vi "from string.vi"(8 "error in":errorcluster, 9 "data":string, 10 "version":string, 11 "user tag bus module configuration In":refnum<class "user tag bus module configuration.lvclass">) -> (0 "error out":errorcluster, 3 "user tag bus module configuration Out":refnum<class "user tag bus module configuration.lvclass">)   [LabVIEW 2013, in "user tag bus module configuration.lvclass"]
doc: "Provides an interface for loading a module configuration from a file or other serialized data source. It is recommended that all children of this class store data in two sets--data required for its own initialization, and any data required for parent initialization--and that each implementation uses the <b>Call Parent Method</b> primitive to de-serialize parent information. As a result, it is expected that every module configuration class calls <b>component configuration.lvclass:From String.vi</b>."
uses:
  user tag bus module configuration.lvclass
  state module configuration.ctl
  <vilib>/NI/Tag Bus Module Framework/channel/TBM channel.lvclass
  control module configuration.ctl
  gains.ctl
  <vilib>/NI/Tag Bus Module Framework/module configuration/TBM module configuration.lvclass
  user tag bus module configuration.lvclass/user tag bus module configuration.ctl
  <vilib>/NI/Tag Bus Module Framework/root configuration/wrap data.vi
  <vilib>/NI/Tag Bus Module Framework/root configuration/create GUID.vi
  <vilib>/NI/Tag Bus Module Framework/root configuration/TBM configuration.lvclass
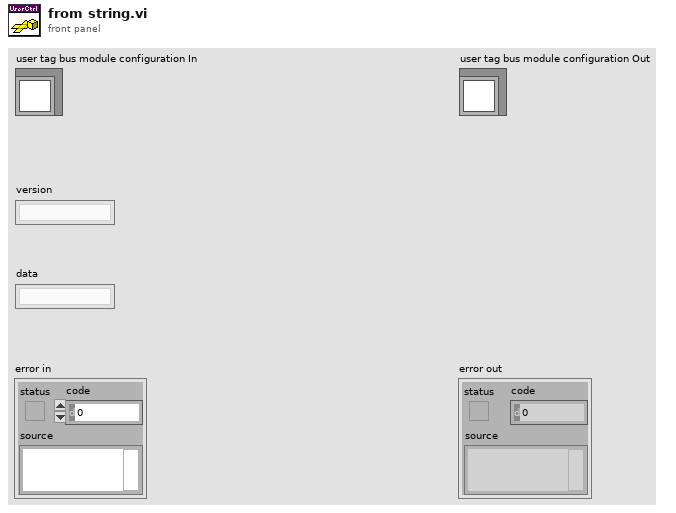
[diagram p1: front panel]
types:
  T1 = typedef "user tag bus module configuration.lvclass/control module configuration.ctl" = cluster{"name":string, "setpoint":refnum<class "TBM channel.lvclass">, "process variable":refnum<class "TBM channel.lvclass">, "output":refnum<class "TBM channel.lvclass">, "gains":T2, "output range":cluster{"output high":dbl, "output low":dbl}}
  T2 = typedef "user tag bus module configuration.lvclass/gains.ctl" = cluster{"Kp":dbl, "Ki":dbl, "Kd":dbl}
  T3 = typedef "user tag bus module configuration.lvclass/state module configuration.ctl" = cluster{"fixed input":refnum<class "TBM channel.lvclass">, "fixed output":refnum<class "TBM channel.lvclass">, "initial state":u8}
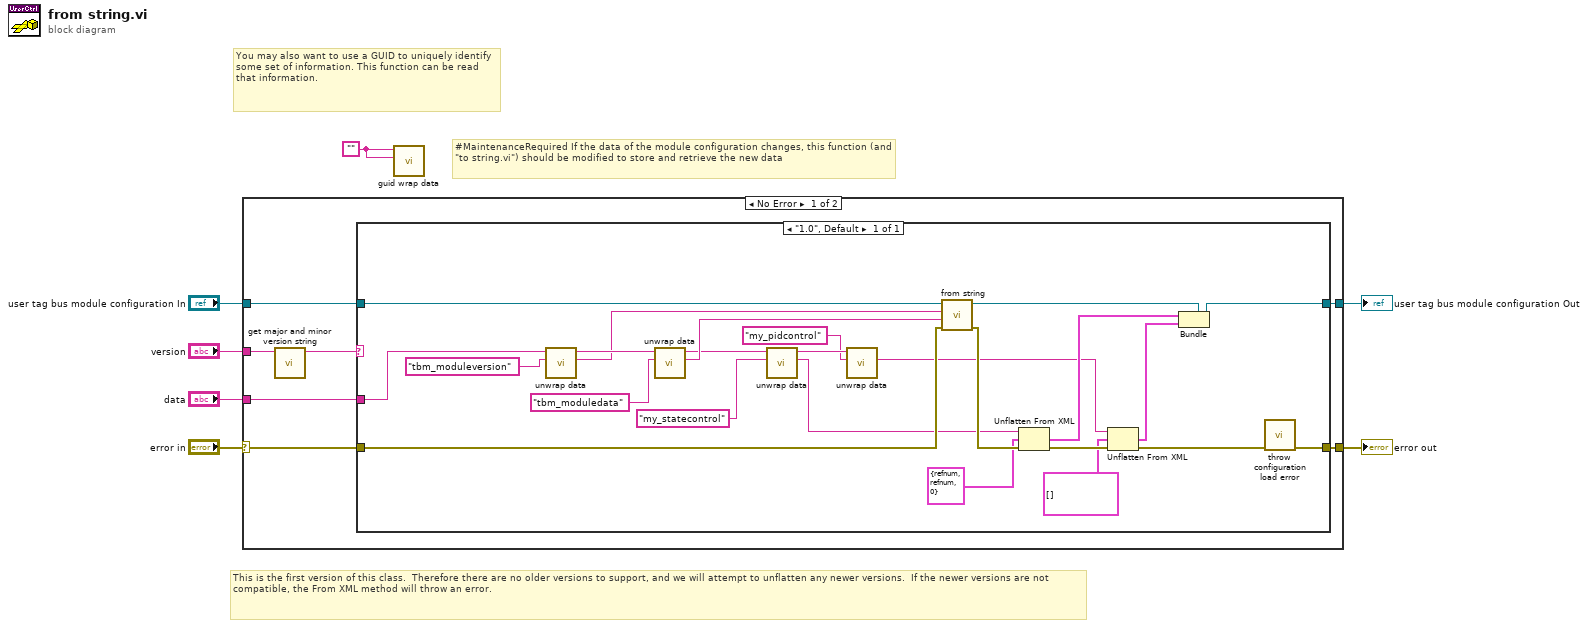
[diagram p0: block diagram]
diagram:
  w1 = ""
  # "You may also want to use a GUID to uniquely identify some set of information. This function can be read that information."
  # "#MaintenanceRequired If the data of the module configuration changes, this function (and \"to string.vi\") should be modified to store and retrieve the new data"
  # "This is the first version of this class.  Therefore there are no older versions to support, and we will attempt to unflatten any newer versions.  If the newer versions are not compatible, the From XML method will throw an error."
  n1 = case shown="No Error" "error in" {
    selector: "error in" -> [w8 w40]
    tunnel: "data" -> [w14 _]
    tunnel: "user tag bus module configuration In" -> [w13 w39]
    tunnel: [w12 w39] -> w6
    tunnel: [w11 w40] -> w5
    tunnel: "version" -> [w10 _]
    frame No Error {
      n2 = call <vilib>:"get major and minor version string.vi"("full version"=w10) -> ("major.minor version"=w9:string)  [unwired: 10 in]
      n3 = case shown="\"1.0\", Default" w9 {
        tunnel: w14 -> [w33]
        tunnel: w8 -> [w32]
        tunnel: w13 -> [w38]
        tunnel: [w27] -> w12
        tunnel: [w35] -> w11
        frame "1.0", Default {
          n4 = call <vilib>:"unwrap data.vi"("identifier"="tbm_moduleversion" ("additional identifier"), "data to unwrap"=w33) -> ("unwrapped data"=w28:string, "remaining string"=w34:string)  [unwired: 8 in]
          n5 = call <vilib>:"unwrap data.vi"("identifier"="tbm_moduledata" ("additional identifier"), "data to unwrap"=w34) -> ("unwrapped data"=w30:string, "remaining string"=w25:string)  [unwired: 8 in]
          n6 = call <vilib>:"unwrap data.vi"("identifier"="my_statecontrol" ("additional identifier"), "data to unwrap"=w25) -> ("unwrapped data"=w23:string, "remaining string"=w17:string)  [unwired: 8 in]
          n7 = call <vilib>:"unwrap data.vi"("identifier"="my_pidcontrol" ("additional identifier"), "data to unwrap"=w17) -> ("unwrapped data"=w15:string)  [unwired: 8 in, 1 out]
          n8 = call-parent "from string.vi"("error in"=w32, "data"=w30, "version"=w28, "module configuration in"=w38) -> ("error out"=w36:errorcluster, "module configuration out"=w37:refnum<class "user tag bus module configuration.lvclass">)  [unwired: 6 in]
          n9 = Unflatten From XML(xml string=w23, type=T3 {"fixed input"=refnum, "fixed output"=refnum, "initial state"=0} ("state module configuration"), error in (no error)=w36) -> (value=w20:T3, error out=w26:errorcluster)
          n10 = Unflatten From XML(xml string=w15, type=T1[] [] ("control functions"), error in (no error)=w26) -> (value=w18:T1[], error out=w22:errorcluster)
          n11 = Bundle(cluster=w37, w20, w18) -> (w27:refnum<class "user tag bus module configuration.lvclass">)
          n12 = call <vilib>:"throw configuration load error.vi"("error in"=w22) -> ("error out"=w35:errorcluster)  [unwired: 10 in]
        }
      }
    }
    frame Error {
    }
  }
  "error out" <- w5
  "user tag bus module configuration Out" <- w6
  n13 = call <vilib>:"guid wrap data.vi"("identifier"=w1, "data to wrap"=w1) -> ()  [unwired: 8 in, 2 out]
